vi "sub_take_measurements.vi"(8 "error in (no error)":errorcluster, 10 "Live data in":T1, 11 "Input parameters":T2={"Measurement type"=enum."Debug", "Sensor type"=enum."HPK_8in_256ch", "Identifier"="test.txt", "Open after execution?"=FALSE, "Plot after execution?"=FALSE, "Display channel"=0, "Voltage Delay (s)"=0.5, "Switch Delay (s)"=0.01, "VISA resource name source"="", "VISA resource name DMM"="", "VISA resource name LCR"="", "Compliance  Level (A)"=10.0, "Voltage Limit (V)"=1000.0, "Data storage location"="", "Scan voltages"="", "Use source as DMM?"=FALSE, "LCR signal frequenzy (Hz)"=10.0, "DMM device"=enum."Keithley2001", "Sampling number"=1, "Use env. sensors on"=enum."Sensirion sht1x/7x", "Switchboard Handle"=0, "Use Switchboard"=FALSE, "LCR signal voltage (V)"=10000.0, "Repeat"=1, "Scan voltages IV"="", "Scan voltages CV"="", "Hex pad numbers?"=FALSE, "Set measurement type"=enum."Debug", "Custom pad scan"="", "IV voltage Delay (s)"=0.5, "CV voltage Delay (s)"=0.5, "Needle measurement?"=FALSE, "Comments"="test.txt", "LCR signal frequenzy (kHz)"=10.0, "Compliance  Level (uA)"=10.0, "Open Correction Array"=array2304x3[6912 elements], "Current set voltage"=0.0, "Last set voltage"=0.0, "Current channel"=0, "Last OpenCorrection index"=-1, "Total curr/vltg every x steps"=10, "Current channel iteration"=0, "No CV corrections"=FALSE, "Mapfile"="", "Corrfile"="", "IV voltage file"=path "", "CV voltage file"=path "", "IV Switch Delay (s)"=0.01, "CV Switch Delay (s)"=0.01, "Invert polarity"=FALSE, "Set debug dirs"=FALSE, "Is n on p"=FALSE} {"CV Switch Delay (s)" format="%#_13g"; "IV Switch Delay (s)" format="%#_13g"; "Last set voltage" format="%#_13g"; "Current set voltage" format="%#_13g"; "CV voltage Delay (s)" format="%#_13g"; "IV voltage Delay (s)" format="%#_13g"; "Voltage Limit (V)" format="%#_13g"; "Voltage Delay (s)" format="%#_13g"; "Switch Delay (s)" format="%#_13g"}) -> (0 "error out":errorcluster, 2 "Live data out":T1, 3 "Input parameters out":T2={"Measurement type"=enum."Debug", "Sensor type"=enum."HPK_8in_256ch", "Identifier"="test.txt", "Open after execution?"=FALSE, "Plot after execution?"=FALSE, "Display channel"=0, "Voltage Delay (s)"=0.5, "Switch Delay (s)"=0.01, "VISA resource name source"="", "VISA resource name DMM"="", "VISA resource name LCR"="", "Compliance  Level (A)"=10.0, "Voltage Limit (V)"=1000.0, "Data storage location"="", "Scan voltages"="", "Use source as DMM?"=FALSE, "LCR signal frequenzy (Hz)"=10.0, "DMM device"=enum."Keithley2001", "Sampling number"=1, "Use env. sensors on"=enum."Sensirion sht1x/7x", "Switchboard Handle"=0, "Use Switchboard"=FALSE, "LCR signal voltage (V)"=10000.0, "Repeat"=1, "Scan voltages IV"="", "Scan voltages CV"="", "Hex pad numbers?"=FALSE, "Set measurement type"=enum."Debug", "Custom pad scan"="", "IV voltage Delay (s)"=0.5, "CV voltage Delay (s)"=0.5, "Needle measurement?"=FALSE, "Comments"="test.txt", "LCR signal frequenzy (kHz)"=10.0, "Compliance  Level (uA)"=10.0, "Open Correction Array"=array2304x3[6912 elements], "Current set voltage"=0.0, "Last set voltage"=0.0, "Current channel"=0, "Last OpenCorrection index"=-1, "Total curr/vltg every x steps"=10, "Current channel iteration"=0, "No CV corrections"=FALSE, "Mapfile"="", "Corrfile"="", "IV voltage file"=path "", "CV voltage file"=path "", "IV Switch Delay (s)"=0.01, "CV Switch Delay (s)"=0.01, "Invert polarity"=FALSE, "Set debug dirs"=FALSE, "Is n on p"=FALSE} {"CV Switch Delay (s)" format="%#_13g"; "IV Switch Delay (s)" format="%#_13g"; "Last set voltage" format="%#_13g"; "Current set voltage" format="%#_13g"; "CV voltage Delay (s)" format="%#_13g"; "IV voltage Delay (s)" format="%#_13g"; "Voltage Limit (V)" format="%#_13g"; "Voltage Delay (s)" format="%#_13g"; "Switch Delay (s)" format="%#_13g"}, 4 "Compliance reached?":bool)   [LabVIEW 2016]
doc: "Handles the device readout for a single measurement (one pad, one voltage)"
uses:
  input_params.ctl
  data_live.ctl
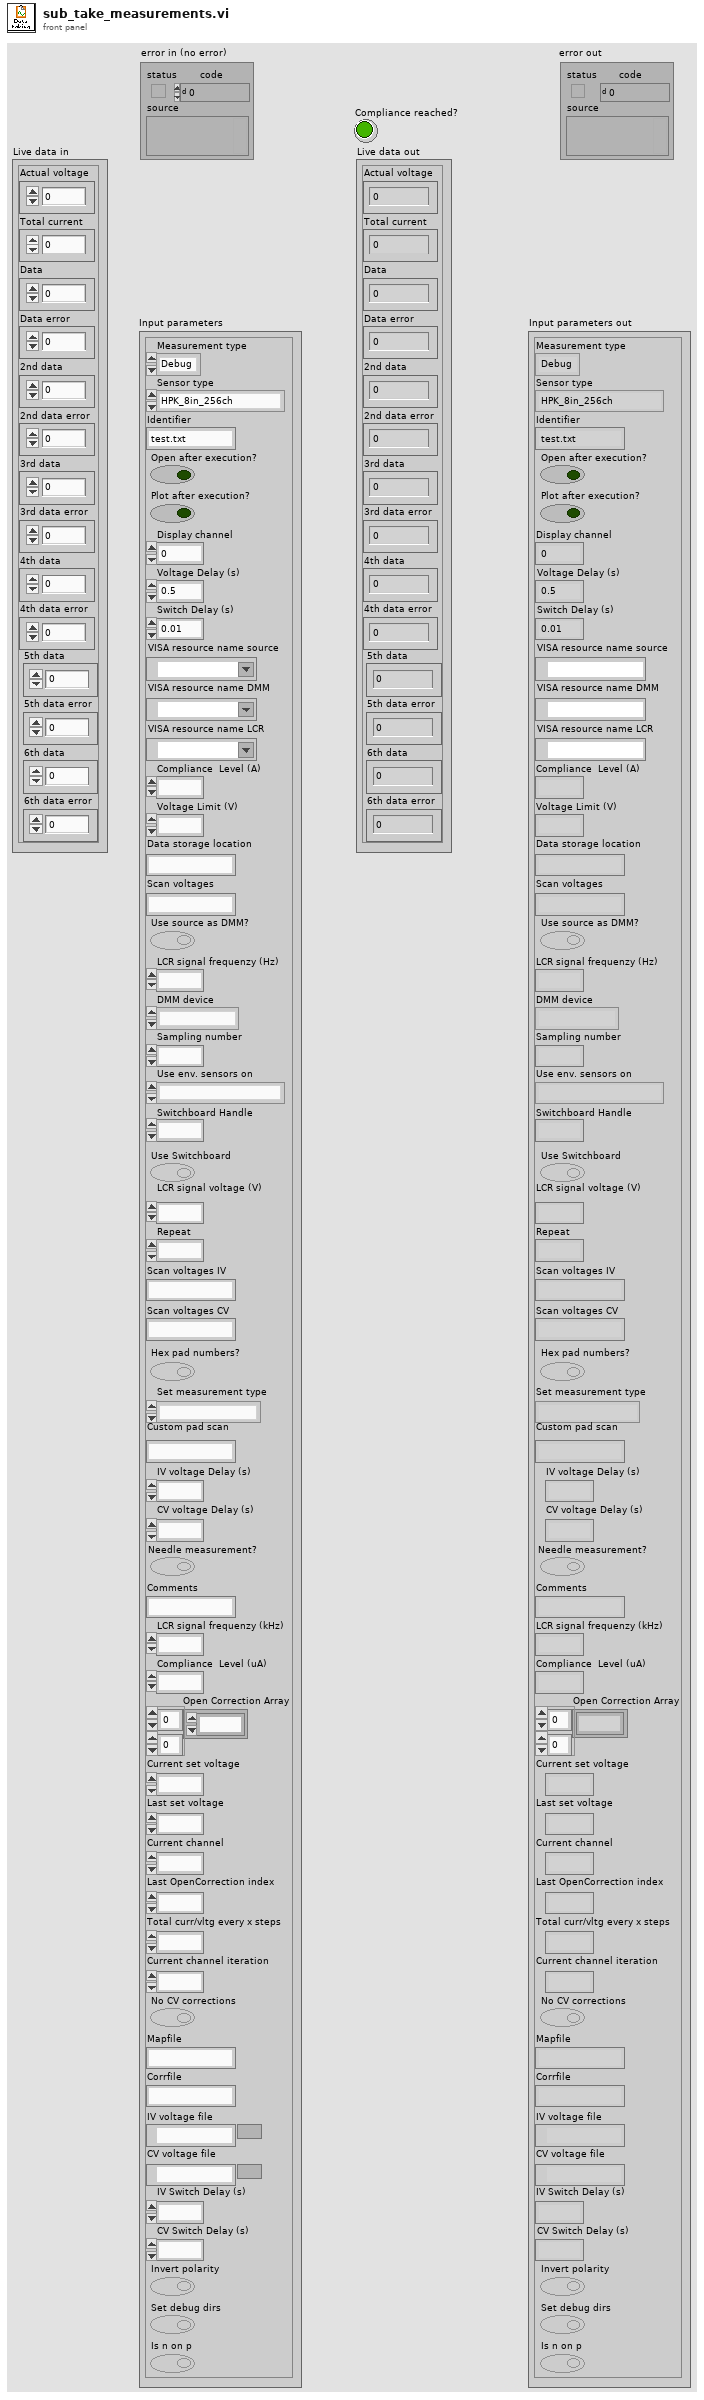
[diagram p1: front panel]
types:
  T1 = typedef "data_live.ctl" = cluster{"Actual voltage":dbl, "Total current":dbl, "Data":dbl, "Data error":dbl, "2nd data":dbl, "2nd data error":dbl, "3rd data":dbl, "3rd data error":dbl, "4th data":dbl, "4th data error":dbl, "6th data error":dbl, "6th data":dbl, "5th data error":dbl, "5th data":dbl}
  T2 = typedef "input_params.ctl" = cluster{"Measurement type":enum16{"IV", "CV", "Debug", "Test_contact"}, "Sensor type":enum16{"HPK_6in_135ch", "HPK_8in_256ch", "IFX_8in_256ch", "Diode", "HPK_6in_256ch", "Full_Matrix", ""}, "Identifier":string, "Open after execution?":bool, "Plot after execution?":bool, "Display channel":i32, "Voltage Delay (s)":dbl, "Switch Delay (s)":dbl, "VISA resource name source":refnum<visa-resource-name>, "VISA resource name DMM":refnum<visa-resource-name>, "VISA resource name LCR":refnum<visa-resource-name>, "Compliance  Level (A)":dbl, "Voltage Limit (V)":dbl, "Data storage location":string, "Scan voltages":string, "Use source as DMM?":bool, "LCR signal frequenzy (Hz)":dbl, "DMM device":enum16{"Keithley2001", "Keithley2450", "Keithley2410", "Keithley6487", "Keithley6517"}, "Sampling number":i32, "Use env. sensors on":enum16{"Sensirion sht1x/7x", "Switch Matrix", "Probecard"}, "Switchboard Handle":u32, "Use Switchboard":bool, "LCR signal voltage (V)":dbl, "Repeat":i32, "Scan voltages IV":string, "Scan voltages CV":string, "Hex pad numbers?":bool, "Set measurement type":enum16{"IV", "CV", "Debug", "Test_contact", "IV+CV"}, "Custom pad scan":string, "IV voltage Delay (s)":dbl, "CV voltage Delay (s)":dbl, "Needle measurement?":bool, "Comments":string, "LCR signal frequenzy (kHz)":dbl, "Compliance  Level (uA)":dbl, "Open Correction Array":dbl[][], "Current set voltage":dbl, "Last set voltage":dbl, "Current channel":i32, "Last OpenCorrection index":i32, "Total curr/vltg every x steps":i32, "Current channel iteration":i32, "No CV corrections":bool, "Mapfile":string, "Corrfile":string, "IV voltage file":path, "CV voltage file":path, "IV Switch Delay (s)":dbl, "CV Switch Delay (s)":dbl, "Invert polarity":bool, "Set debug dirs":bool, "Is n on p":bool}
  T3 = typedef "data_LCR.ctl" = cluster{"Z":dbl, "Z error":dbl, "Theta":dbl, "Theta error":dbl, "Cp uncorrected [pF]":dbl, "Cp uncorrected error [pF]":dbl, "Cp [pF]":dbl, "Cp error [pF]":dbl, "Cs [pF]":dbl, "Cs error [pF]":dbl, "Cs uncorrected [pF]":dbl, "Cs uncorrected error [pF]":dbl}
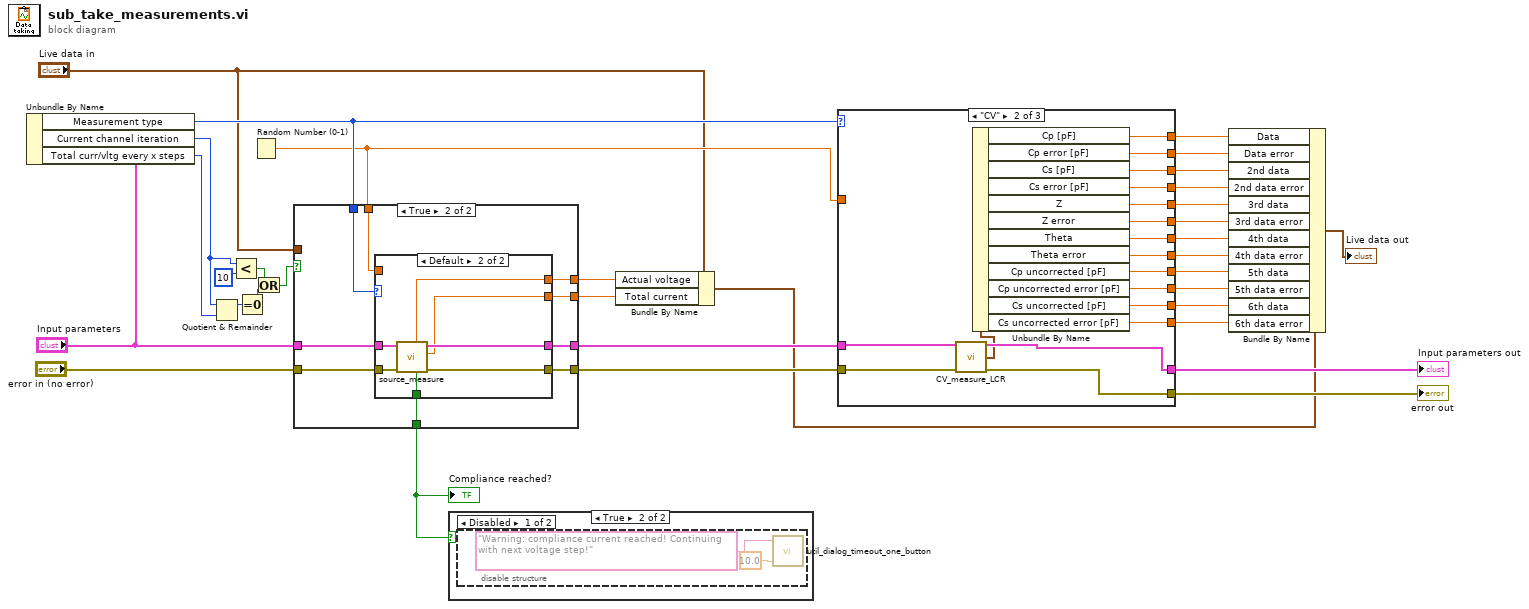
[diagram p0: block diagram]
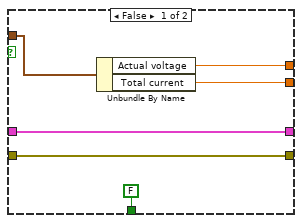
[diagram p2: hidden frame]
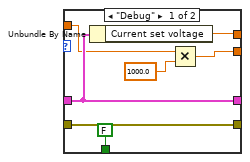
[diagram p3: hidden frame]
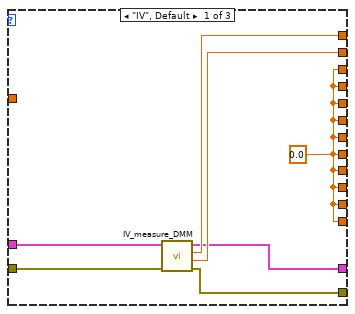
[diagram p6: hidden frame]
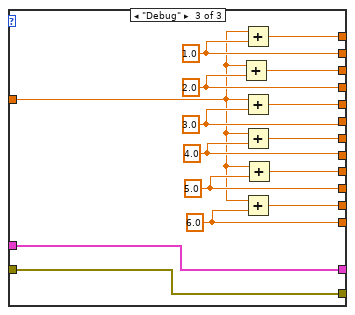
[diagram p7: hidden frame]
diagram:
  n1 = Unbundle By Name("Input parameters") -> ("Measurement type"=w13:enum16{"IV", "CV", "Debug", "Test_contact"}, "Current channel iteration"=w2:i32, "Total curr/vltg every x steps"=w8:i32)
  n2 = Quotient & Remainder(x=w2, y=w8) -> (x-y*floor(x/y)=w7:i32)  [unwired: 1 out]
  n3 = Less?(x=w2, y=10) -> (x < y?=w5:bool)
  n4 = Equal To 0?(x=w7) -> (x = 0?=w4:bool)
  n5 = Random Number (0-1)() -> (number: 0 to 1=w9:dbl)
  n6 = Or(x=w5, y=w4) -> (x .or. y?=w3:bool)
  n7 = case shown="True" w3 {
    tunnel: "Input parameters" -> [w36 w48]
    tunnel: [w36 w47] -> w17
    tunnel: "error in (no error)" -> [w35 w46]
    tunnel: [w35 w45] -> w15
    tunnel: [FALSE ("Compliance reached?") w44] -> w14
    tunnel: w13 -> [_ w43]
    tunnel: [w38 w42] -> w11
    tunnel: [w37 w41] -> w10
    tunnel: w9 -> [_ w40]
    tunnel: "Live data in" -> [w39 _]
    frame False {
      n8 = Unbundle By Name(w39) -> ("Actual voltage"=w38:dbl, "Total current"=w37:dbl)
    }
    frame True {
      n9 = case shown="Default" w43 {
        tunnel: w48 -> [w53 w62]
        tunnel: [w53 w61] -> w47
        tunnel: w46 -> [w55 w60]
        tunnel: [w55 w59] -> w45
        tunnel: [FALSE ("Compliance reached?") w58] -> w44
        tunnel: [w52 w57] -> w42
        tunnel: [w49 w56] -> w41
        tunnel: w40 -> [w50 _]
        frame "Debug" {
          n10 = Unbundle By Name(w53) -> ("Current set voltage"=w52:dbl)
          n11 = Multiply(x=w50, y=1000.0 ("number: 0 to 1")) -> (x*y=w49:dbl)
        }
        frame Default {
          n12 = call "source_measure.vi"("error in (no error)"=w60, "Input parameters"=w62) -> ("error out"=w59:errorcluster, "Total current"=w56:dbl, "Input parameters"=w61:T2, "Compliance reached?"=w58:bool, "Actual voltage"=w57:dbl)  [unwired: 5 in]
        }
      }
    }
  }
  "Compliance reached?" <- w14
  n13 = case shown="True" w14 {
    frame False {
    }
    frame True {
      n14 = disable-structure shown="Disabled" {
        frame Disabled {
          n15 = call "util_dialog_timeout_one_button.vi"("Message text"="Warning: compliance current reached! Continuing with next voltage step!", "Timeout (s)"=10.0) -> ()  [unwired: 4 in]
        }
        frame Enabled {
        }
      }
    }
  }
  n16 = Bundle By Name(cluster="Live data in", "Actual voltage"=w11, "Total current"=w10) -> (w12:T1)
  n17 = case shown="\"CV\"" w13 {
    tunnel: [w69 w86 w100] -> w30
    tunnel: w15 -> [w66 w73 w103]
    tunnel: [w71 w88 w103] -> w32
    tunnel: [w67 w84 w98] -> w27
    tunnel: [w67 w82 w96] -> w26
    tunnel: [w67 w81 w94] -> w25
    tunnel: w17 -> [w65 w72 w102]
    tunnel: [w70 w85 w101] -> w29
    tunnel: [w67 w83 w99] -> w28
    tunnel: [w67 w80 w97] -> w24
    tunnel: [w67 w79 w95] -> w23
    tunnel: [w68 w87 w102] -> w33
    tunnel: [w67 w77 w92] -> w22
    tunnel: [w67 w76 w91] -> w21
    tunnel: [w67 w75 w93] -> w20
    tunnel: [w67 w74 w90] -> w19
    tunnel: w9 -> [_ _ w89]
    frame "IV", Default {
      w67 = 0.0 ("Secondary Parameter")
      n18 = call "IV_measure_DMM.vi"("error in (no error)"=w66, "Input parameters"=w65) -> ("error out"=w71:errorcluster, "Error"=w70:dbl, "Result"=w69:dbl, "Input parameters out"=w68:T2)  [unwired: 6 in]
    }
    frame "CV" {
      n19 = call "CV_measure_LCR.vi"("Input parameters"=w72, "error in (no error)"=w73) -> ("Input parameters out"=w87:T2, "LCR data"=w78:T3, "error out"=w88:errorcluster)  [unwired: 11 in]
      n20 = Unbundle By Name(w78) -> ("Cp [pF]"=w86:dbl, "Cp error [pF]"=w85:dbl, "Cs [pF]"=w84:dbl, "Cs error [pF]"=w83:dbl, "Z"=w82:dbl, "Z error"=w80:dbl, "Theta"=w81:dbl, "Theta error"=w79:dbl, "Cp uncorrected [pF]"=w77:dbl, "Cp uncorrected error [pF]"=w76:dbl, "Cs uncorrected [pF]"=w75:dbl, "Cs uncorrected error [pF]"=w74:dbl)
    }
    frame "Debug" {
      w90 = 6.0 ("y")
      w91 = 5.0 ("y")
      w101 = 1.0 ("y")
      w99 = 2.0 ("y")
      w97 = 3.0 ("y")
      w95 = 4.0 ("y")
      n21 = Add(x=w89, y=w99) -> (x+y=w98:dbl)
      n22 = Add(x=w89, y=w101) -> (x+y=w100:dbl)
      n23 = Add(x=w89, y=w97) -> (x+y=w96:dbl)
      n24 = Add(x=w89, y=w95) -> (x+y=w94:dbl)
      n25 = Add(x=w89, y=w90) -> (x+y=w93:dbl)
      n26 = Add(x=w89, y=w91) -> (x+y=w92:dbl)
    }
  }
  "Input parameters out" <- w33
  "error out" <- w32
  n27 = Bundle By Name(cluster=w12, "Data"=w30, "Data error"=w29, "2nd data"=w27, "2nd data error"=w28, "3rd data"=w26, "3rd data error"=w24, "4th data"=w25, "4th data error"=w23, "5th data"=w22, "5th data error"=w21, "6th data"=w20, "6th data error"=w19) -> (→"Live data out":T1)
